vi "Merge gRPC Error.vi"(8 "error in (no error)":errorcluster, 10 "gRPC Error":T1) -> (0 "error out":errorcluster)   [LabVIEW 2021, in "CIFPluginLoaderClientWrapper.lvlib"]
uses:
  CIFPluginLoaderClientWrapper.lvlib
  CIF_PluginLoader_client/RPC Messages/cif_common_Status.ctl
  CIF_PluginLoader_client/CIF_PluginLoader_client.lvlib
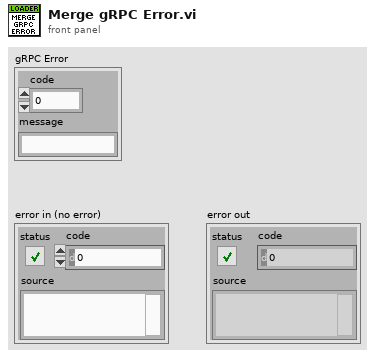
[diagram p1: front panel]
types:
  T1 = typedef "CIF_PluginLoader_client.lvlib/cif_common_Status.ctl" = cluster{"code":i32, "message":string}
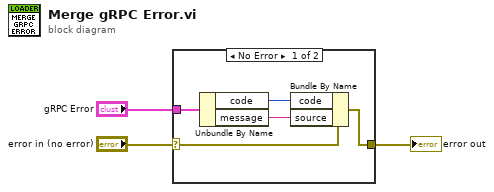
[diagram p0: block diagram]
diagram:
  n1 = case shown="No Error" "error in (no error)" {
    selector: "error in (no error)" -> [w7 w9]
    tunnel: [w4 w9] -> w2
    tunnel: "gRPC Error" -> [w8 _]
    frame No Error {
      n2 = Unbundle By Name(w8) -> ("code"=w6:i32, "message"=w5:string)
      n3 = Bundle By Name(cluster=w7, "code"=w6, "source"=w5) -> (w4:errorcluster)
    }
    frame Error {
    }
  }
  "error out" <- w2
